vi "ConfFileParser.vi"(0 "TEXT":string, 1 "search Indexes array":string[](array[string])) -> (2 "Cluster Array":cluster{"trimmed string":string, "Num":i32}[](array[cluster]), 3 "Names":string[](array[string]), 4 "Codes":i32[](array[numeric]))   [LabVIEW 2010]
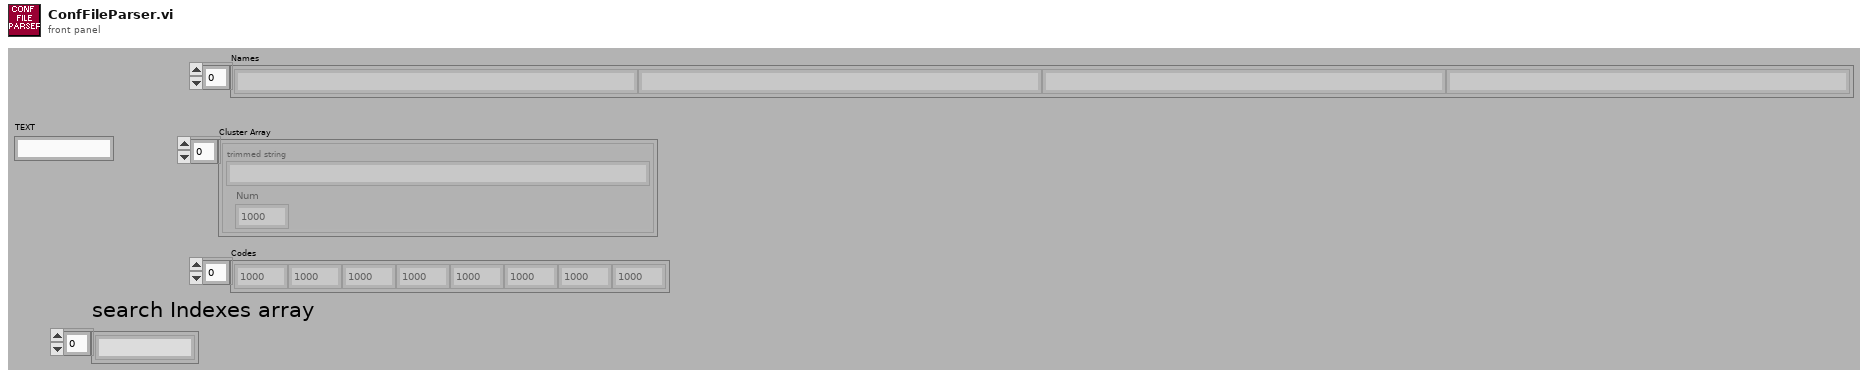
[diagram p1: front panel]
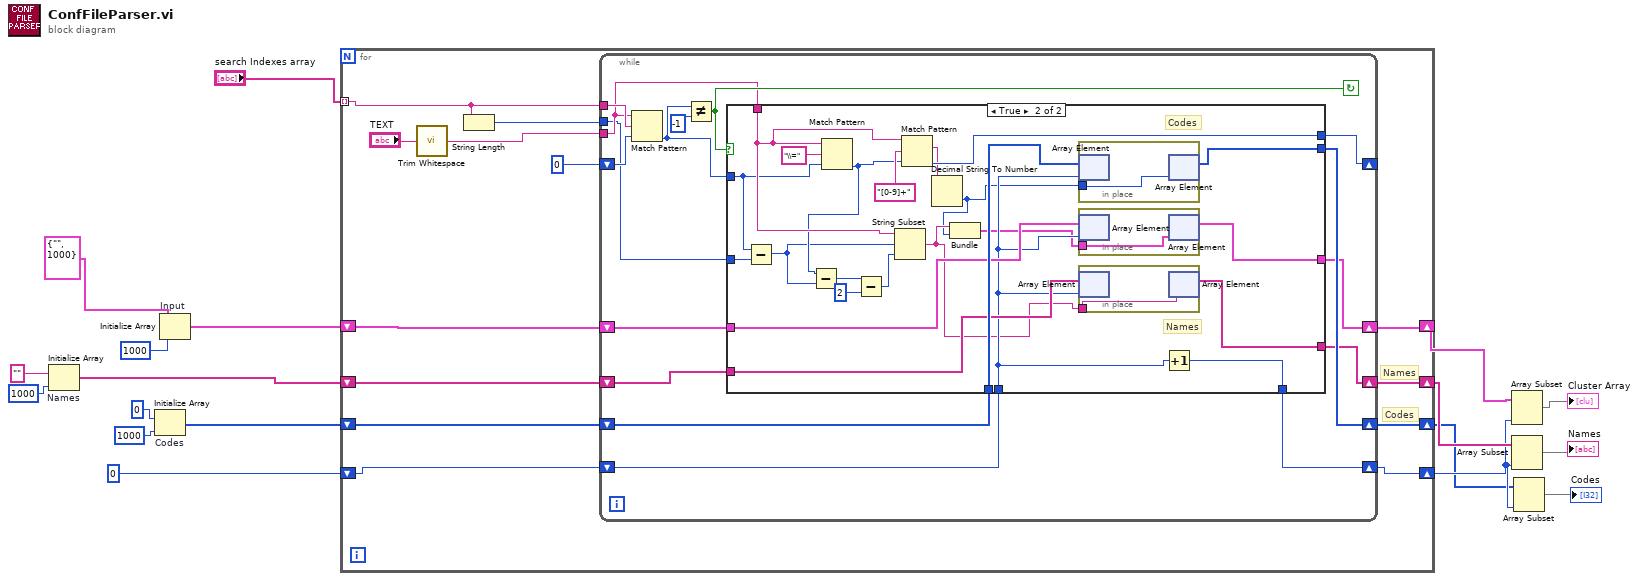
[diagram p0: block diagram]
diagram:
  n1 = Initialize Array "Names"("" ("trimmed string"), 1000 ("dimension size")) -> (w8:string[])
  n2 = Initialize Array "Codes"(0 ("dimension size"), 1000 ("dimension size")) -> (w14:i32[])
  n3 = Initialize Array "Input"(cluster{"trimmed string":string, "Num":i32} {"trimmed string"="", "Num"=1000} ("output cluster"), 1000 ("dimension size")) -> (w4:cluster{"trimmed string":string, "Num":i32}[])
  n4 = for {
    tunnel: "search Indexes array" -> [w20] mode=indexing
    shift-right: [w19] -> w1
    shift-left: w4 -> [w21]
    shift-right: [w25] -> w12
    shift-left: w8 -> [w22]
    shift-right: [w23] -> w9
    shift-left: w14 -> [w28]
    shift-right: [w24] -> w10
    shift-left: 0 ("dimension size") -> [w26]
    # "Names"
    # "Codes"
    n5 = call <vilib>:"Trim Whitespace.vi"("string"="TEXT") -> ("trimmed string"=w30:string)  [unwired: 1 in]
    n6 = String Length(string=w20) -> (length=w27:i32)
    n7 = while {
      tunnel: w20 -> [w45]
      tunnel: w30 -> [w43]
      shift-right: [w38] -> _
      shift-left: 0 ("offset (0)") -> [w40]
      shift-right: [w35] -> w19
      shift-left: w21 -> [w36]
      shift-right: [w32] -> w25
      shift-left: w22 -> [w34]
      shift-right: [w41] -> w23
      shift-left: w28 -> [w42]
      tunnel: w27 -> [w39]
      shift-right: [w33] -> w24
      shift-left: w26 -> [w37]
      stop <- w46 continue-if-true
      n8 = Match Pattern(string=w43, regular expression=w45, offset (0)=w40) -> (offset past match=w44:i32)  [unwired: 3 out]
      n9 = Not Equal?(x=w44, y=-1) -> (x != y?=w46:bool)
      n10 = case shown="True" w46 {
        tunnel: w43 -> [_ w73]
        tunnel: w44 -> [w51 w72]
        tunnel: w42 -> [w52 w63]
        tunnel: [w52 w62] -> w41
        tunnel: w39 -> [_ w68]
        tunnel: [w51 w70] -> w38
        tunnel: w37 -> [w50 w57]
        tunnel: w36 -> [w49 w61]
        tunnel: [w49 w60] -> w35
        tunnel: w34 -> [w48 w58]
        tunnel: [w50 w69] -> w33
        tunnel: [w48 w59] -> w32
        frame False {
        }
        frame True {
          # "Names"
          # "Codes"
          n11 = Subtract(x=w72, y=w68) -> (x-y=w67:i32)
          n12 = Match Pattern(string=w73, regular expression="\\=" ("search string"), offset (0)=w72) -> (offset past match=w71:i32)  [unwired: 3 out]
          n13 = Subtract(x=w71, y=w67) -> (x-y=w65:i32)
          n14 = Subtract(x=w65, y=2) -> (x-y=w64:i32)
          n15 = String Subset(string=w73, offset (0)=w67, length (rest)=w64) -> (substring=w55:string)
          n16 = Match Pattern(string=w73, regular expression="[0-9]+", offset (0)=w71) -> (match substring=w56:string, offset past match=w70:i32)  [unwired: 2 out]
          n17 = Decimal String To Number(string=w56) -> (number=w54:i32)  [unwired: 2 in, 1 out]
          n18 = Bundle("trimmed string"=w55, w54) -> (w53:cluster{"trimmed string":string, i32})  [unwired: 1 in]
          n19 = in-place {
            in-place-border: w54 -> [w78]
            n20 = in-place-array #1(w63, w57) -> ()  [unwired: 1 out]
            n21 = in-place-array #1(w78) -> (w62:i32[])  [unwired: 1 out]
          }
          n22 = in-place {
            in-place-border: w53 -> [w77]
            n23 = in-place-array #2(w61, w57) -> ()  [unwired: 1 out]
            n24 = in-place-array #2(w77) -> (w60:cluster{"trimmed string":string, "Num":i32}[])  [unwired: 1 out]
          }
          n25 = in-place {
            in-place-border: w55 -> [w76]
            n26 = in-place-array #3(w58, w57) -> ()  [unwired: 1 out]
            n27 = in-place-array #3(w76) -> (w59:string[])  [unwired: 1 out]
          }
          n28 = Increment(x=w57) -> (x+1=w69:i32)
        }
      }
    }
  }
  n29 = Array Subset(array=w1, length=w10) -> (→"Cluster Array":cluster{"trimmed string":string, "Num":i32}[])  [unwired: 1 in]
  n30 = Array Subset(array=w12, length=w10) -> (→"Names":string[])  [unwired: 1 in]
  n31 = Array Subset(array=w9, length=w10) -> (→"Codes":i32[])  [unwired: 1 in]
